vi "Search by identifier.vi"(10 "Device Info":T1, 11 "array of devices":T2) -> (3 "index of element":i32)   [LabVIEW 2016]
uses:
  Array Device Info.ctl
  Device Info.ctl
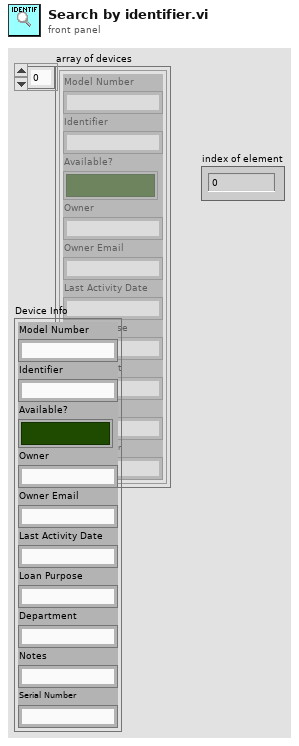
[diagram p1: front panel]
types:
  T1 = typedef "Device Info.ctl" = cluster{"Model Number":string, "Identifier":string, "Available?":bool, "Owner":string, "Owner Email":string, "Last Activity Date":string, "Loan Purpose":string, "Department":string, "Notes":string, "Serial Number":string}
  T2 = typedef "Array Device Info.ctl" = T1[]
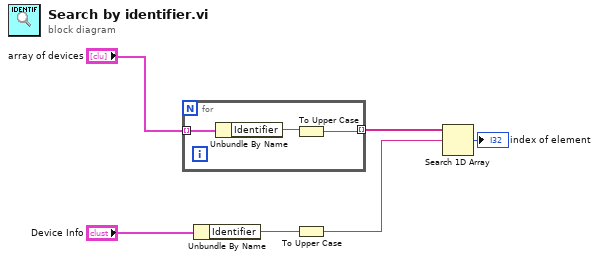
[diagram p0: block diagram]
diagram:
  n1 = for {
    tunnel: "array of devices" -> [w9] mode=indexing
    tunnel: [w7] -> w4 mode=indexing
    n2 = Unbundle By Name(w9) -> ("Identifier"=w8:string)
    n3 = To Upper Case(1:w8) -> (0:w7:string)
  }
  n4 = Unbundle By Name("Device Info") -> ("Identifier"=w2:string)
  n5 = To Upper Case(1:w2) -> (0:w1:string)
  n6 = Search 1D Array(1D array=w4, element=w1) -> (index of element=→"index of element":i32)  [unwired: 1 in]
